vi "To String.vi"(7 "Formatting":enum16{"plain", "fancy"}(ring), 8 "error in":errorcluster, 11 "Vec3d in":refnum<class "Vec3d.lvclass">) -> (0 "error out":errorcluster, 2 "Vec3d String":string, 3 "Vec3d out":refnum<class "Vec3d.lvclass">)   [LabVIEW 2023, in "Vec3d.lvclass"]
uses:
  Vec3d.lvclass
  Vec3d.lvclass/Vec3d.ctl
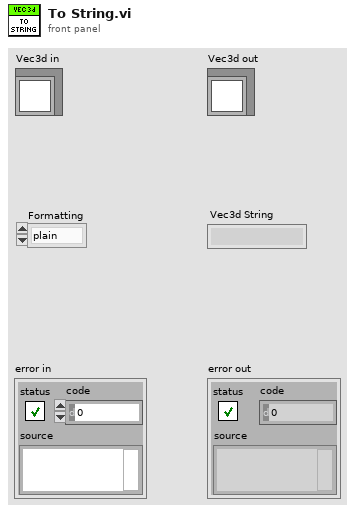
[diagram p1: front panel]
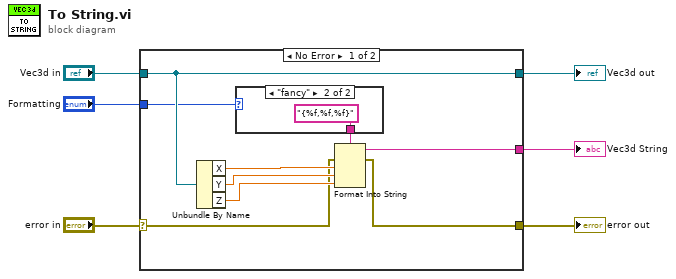
[diagram p0: block diagram]
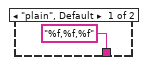
[diagram p2: hidden frame]
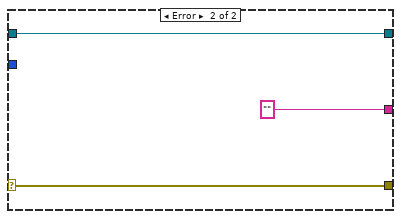
[diagram p3: hidden frame]
diagram:
  n1 = case shown="No Error" "error in" {
    selector: "error in" -> [w10 w20]
    tunnel: [w9 w20] -> w5
    tunnel: [w15 w19] -> w3
    tunnel: "Vec3d in" -> [w15 w19]
    tunnel: [w11 ""] -> w2
    tunnel: "Formatting" -> [w8 _]
    frame No Error {
      n2 = Unbundle By Name(w15) -> ("X"=w14:dbl, "Y"=w13:dbl, "Z"=w12:dbl)
      n3 = case shown="\"fancy\"" w8 {
        tunnel: ["%f,%f,%f" ("format string") "{%f,%f,%f}" ("format string")] -> w7
        frame "plain", Default {
        }
        frame "fancy" {
        }
      }
      n4 = Format Into String(format string=w7, error in=w10, w14, w13, w12) -> (resulting string=w11:string, error out=w9:errorcluster)  [unwired: 1 in]
    }
    frame Error {
    }
  }
  "error out" <- w5
  "Vec3d out" <- w3
  "Vec3d String" <- w2
